vi "XY stage App.vi"() -> ()   [LabVIEW 2017]
uses:
  Newport.XPS.CommandInterface
panel:
  in  "Stop Program":bool
  in  "Start Program":bool
  in  "Move Inverse":bool
  in  "Move Normal":bool
  out "Expected Output":cluster{"X":dbl, "Y":dbl}[](graph)
  out "Total Time Horizontal":dbl
  out "Total Time Vertical":dbl
  in  "Velocity and Acceleration Input":cluster{"Velocity":dbl, "Acceleration":dbl}={"Velocity"=150.0, "Acceleration"=2000.0} {"Acceleration" min=0.0; "Velocity" min=0.0}
  in  "Abort Motion":bool
  out "Total Y Path":dbl
  in  "Absolute Target 2":cluster{"X Position":dbl, "Y Position":dbl}[](array[cluster]) {"Y Position" min=-100.0 max=100.0; "X Position" min=-100.0 max=100.0}
  in  "Start Absolute 2":bool
  out "Current Y Position":dbl[](array[numeric])
  out "Current X Position":dbl[](array[numeric])
  out "Total X Path":dbl
  in  "Number of Horizontal Sections":u32
  in  "Number of Vertical Sections":u32
  in  "Horizontal Segments Parameters":T1(array[cluster]) {"velocity" min=0.0; "Y rel dist" min=-100.0 max=100.0; "X rel dist" min=-100.0 max=100.0}
  in  "Vertical Segments Parameters":T1(array[cluster]) {"velocity" min=0.0; "Y rel dist" min=-100.0 max=100.0; "X rel dist" min=-100.0 max=100.0}
  in  "Absolute Target 1":cluster{"X Position":dbl, "Y Position":dbl}[](array[cluster]) {"Y Position" min=-100.0 max=100.0; "X Position" min=-100.0 max=100.0}
  in  "Start Absolute 1":bool
  in  "Go Home":bool
  in  "Kill All":bool
  # "Absolute Movement"
  # "Relative Movement"
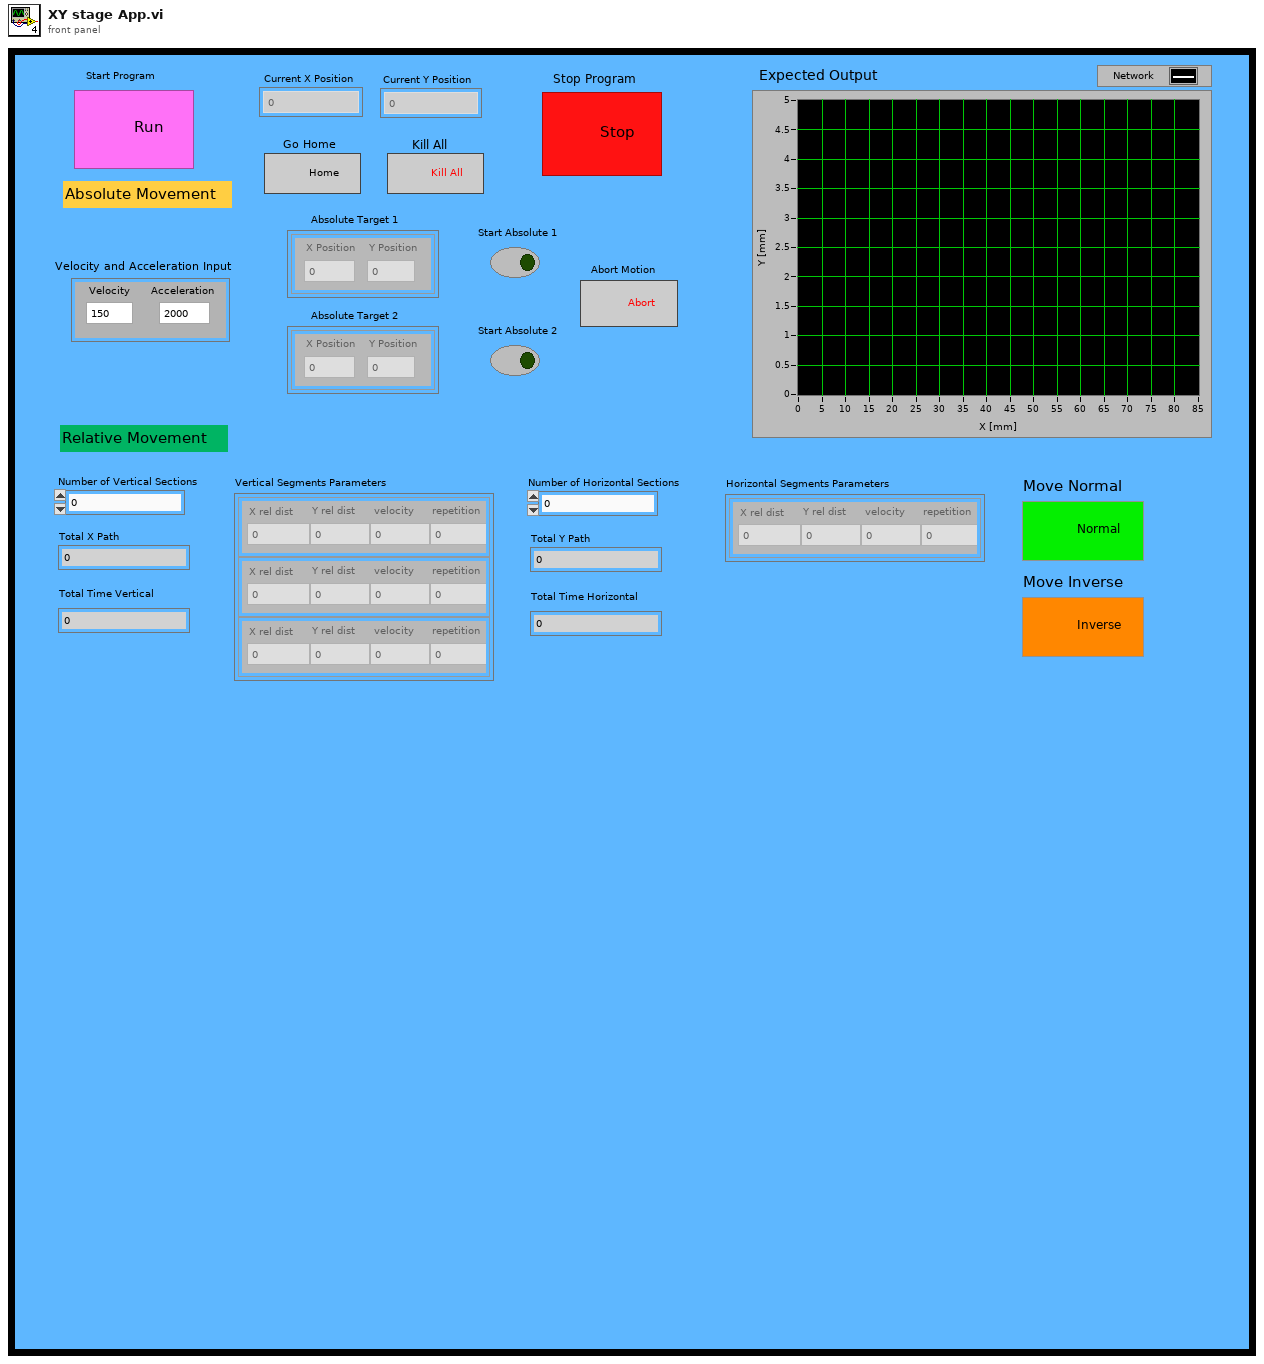
[diagram p1: front panel]
types:
  T1 = cluster{"X rel dist":dbl, "Y rel dist":dbl, "velocity":dbl, "repetition":u32}[]
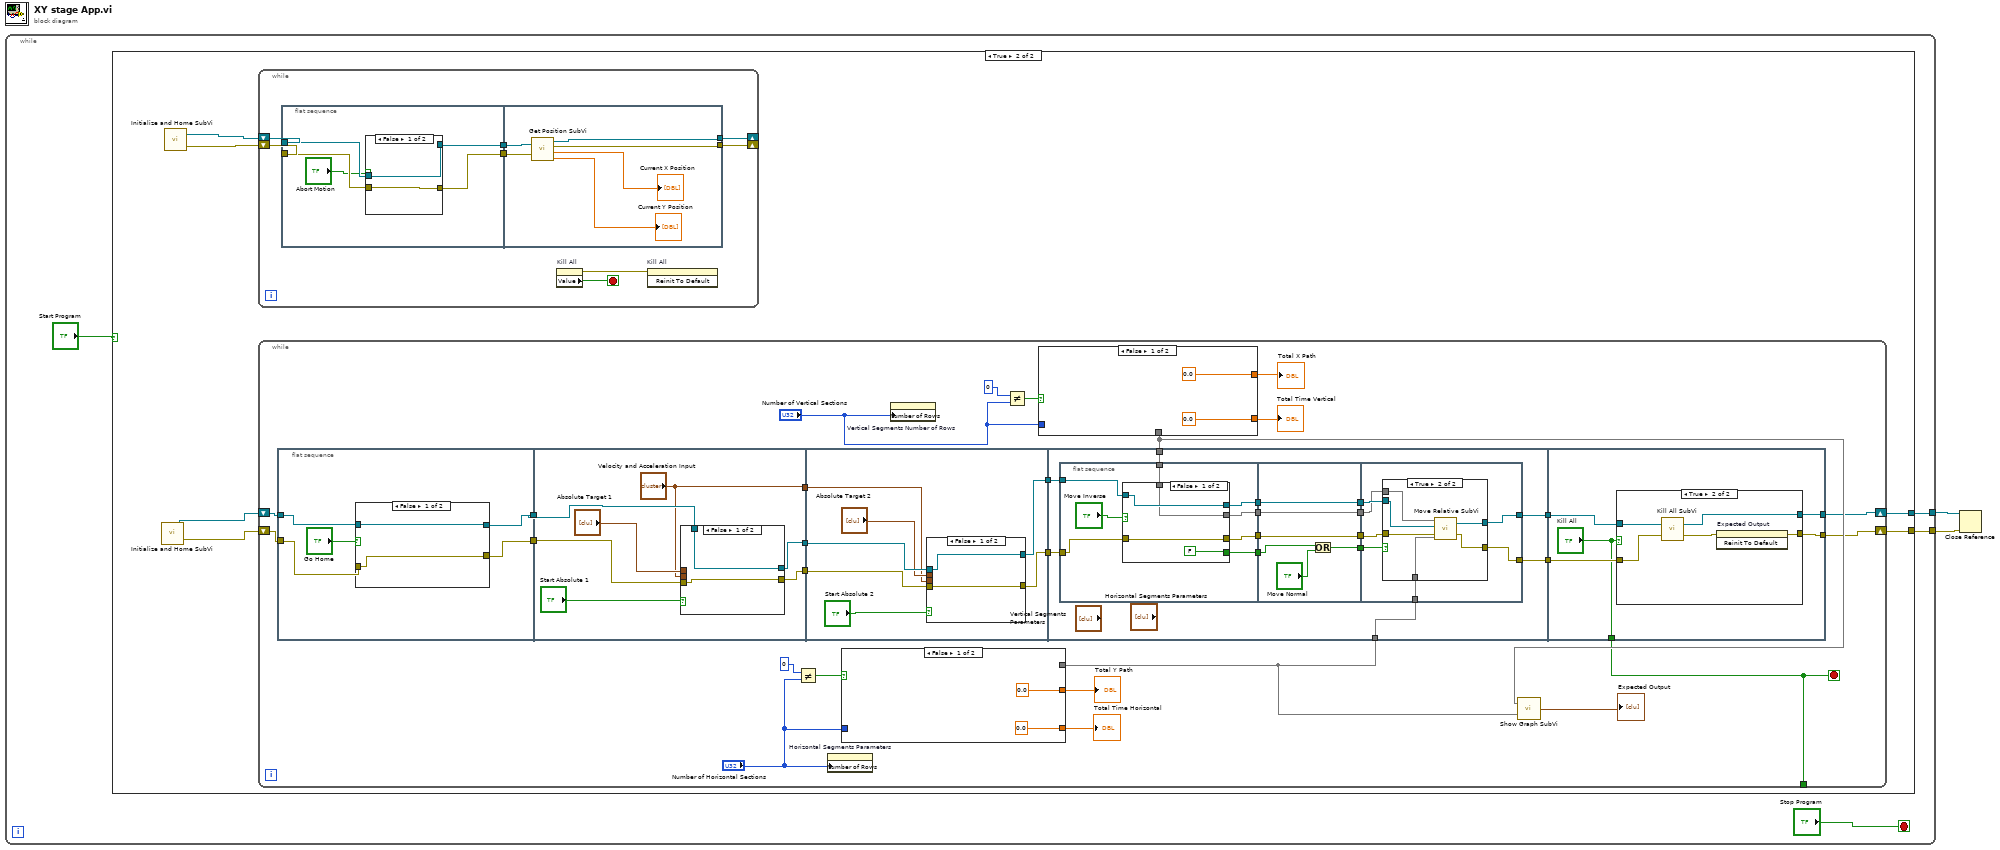
[diagram p0: block diagram]
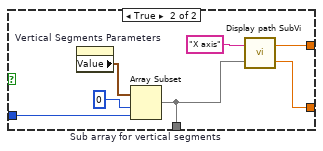
[diagram p3: hidden frame]
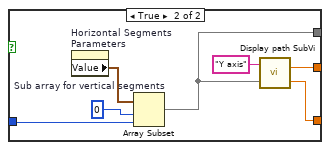
[diagram p4: hidden frame]
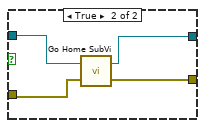
[diagram p5: hidden frame]
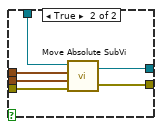
[diagram p6: hidden frame]
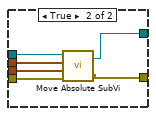
[diagram p7: hidden frame]
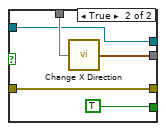
[diagram p8: hidden frame]
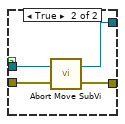
[diagram p11: hidden frame]
diagram:
  n1 = while {
    tunnel: [w6] -> w1
    tunnel: [w5] -> w2
    stop <- "Stop Program" stop-if-true
    n2 = case shown="True" "Start Program" {
      tunnel: [_ w8] -> w6
      tunnel: [_ w7] -> w5
      frame False {
      }
      frame True {
        n3 = call "Initialize and Home SubVi.vi"() -> ("error out"=w11:errorcluster, "reference out"=w12:refnum<k24>)  [unwired: 2 in]
        n4 = call "Initialize and Home SubVi.vi"() -> ("error out"=w9:errorcluster, "reference out"=w10:refnum<k24>)  [unwired: 2 in]
        n5 = while {
          shift-right: [w170] -> _
          shift-left: w10 -> [w168]
          shift-right: [w169] -> _
          shift-left: w9 -> [w167]
          stop <- w164 stop-if-true
          n6 = flat-sequence {
            tunnel: w167 -> [w173]
            tunnel: w168 -> [w174]
            tunnel: [w175] -> w166
            tunnel: [w172] -> w165
            tunnel: [w187] -> w170
            tunnel: [w186] -> w169
            tunnel: w166 -> [w183]
            tunnel: w165 -> [w182]
            frame #0 {
              n7 = case shown="False" "Abort Motion" {
                tunnel: [w177 w180] -> w175
                tunnel: w174 -> [w177 w181]
                tunnel: w173 -> [w176 w179]
                tunnel: [w176 w178] -> w172
                frame False {
                }
                frame True {
                  n8 = call "Abort Move SubVi.vi"("error in"=w179, "reference in"=w181) -> ("error out"=w178:errorcluster, "reference out"=w180:refnum<k24>)
                }
              }
            }
            frame #1 {
              n9 = call "Get Position SubVi.vi"("reference in"=w183, "error in"=w182) -> ("reference out"=w187:refnum<k24>, "error out"=w186:errorcluster, "Current X Position"=→"Current X Position":dbl[], "Current Y Position"=→"Current Y Position":dbl[])
            }
          }
          n10 = property on="Kill All" class="Bool (strict)"() -> (error out=w163:errorcluster, "Value"=w164:bool)  [unwired: 2 in, 1 out]
          n11 = invoke on="Kill All" class="Bool (strict)" method="Reinit To Default"(error in=w163) -> ()  [unwired: 2 in, 3 out]
        }
        n12 = while {
          shift-right: [w15] -> w8
          shift-left: w12 -> [w39]
          shift-right: [w14] -> w7
          shift-left: w11 -> [w38]
          tunnel: [w13] -> _
          stop <- w13 stop-if-true
          n13 = flat-sequence {
            tunnel: w39 -> [w58]
            tunnel: [w59] -> w37
            tunnel: w38 -> [w61]
            tunnel: [w62] -> w36
            tunnel: w37 -> [w75]
            tunnel: w36 -> [w73]
            tunnel: [w71] -> w35
            tunnel: [w70] -> w33
            tunnel: ["Velocity and Acceleration Input"] -> w29
            tunnel: w35 -> [w87]
            tunnel: [w88] -> w34
            tunnel: w33 -> [w90]
            tunnel: [w89] -> w32
            tunnel: w29 -> [w85]
            tunnel: [w101] -> w31
            tunnel: w34 -> [w111]
            tunnel: [w102] -> w30
            tunnel: w32 -> [w110]
            tunnel: w27 -> [w112]
            tunnel: w16 -> [w103]
            tunnel: ["Kill All"] -> w13
            tunnel: w30 -> [w154]
            tunnel: w31 -> [w155]
            tunnel: [w153] -> w15
            tunnel: [w152] -> w14
            frame #0 {
              n14 = case shown="False" "Go Home" {
                tunnel: [w63 w68] -> w62
                tunnel: w61 -> [w63 w67]
                tunnel: [w64 w66] -> w59
                tunnel: w58 -> [w64 w65]
                frame False {
                }
                frame True {
                  n15 = call "Go Home SubVi.vi"("error in"=w67, "reference in"=w65) -> ("error out"=w68:errorcluster, "reference out"=w66:refnum<k24>)
                }
              }
            }
            frame #1 {
              n16 = case shown="False" "Start Absolute 1" {
                tunnel: w75 -> [w76 w83]
                tunnel: "Absolute Target 1" -> [_ w82]
                tunnel: w73 -> [w77 w81]
                tunnel: "Velocity and Acceleration Input" -> [_ w80]
                tunnel: [w76 w79] -> w71
                tunnel: [w77 w78] -> w70
                frame False {
                }
                frame True {
                  n17 = call "Move Absolute SubVi.vi"("error in"=w81, "Vel and Acc"=w80, "Absolute Movement"=w82, "reference in"=w83) -> ("error out"=w78:errorcluster, "reference out"=w79:refnum<k24>)
                }
              }
            }
            frame #2 {
              n18 = case shown="False" "Start Absolute 2" {
                tunnel: w90 -> [w91 w98]
                tunnel: [w91 w97] -> w89
                tunnel: [w92 w96] -> w88
                tunnel: w87 -> [w92 w95]
                tunnel: "Absolute Target 2" -> [_ w94]
                tunnel: w85 -> [_ w93]
                frame False {
                }
                frame True {
                  n19 = call "Move Absolute SubVi.vi"("error in"=w98, "Vel and Acc"=w93, "Absolute Movement"=w94, "reference in"=w95) -> ("error out"=w97:errorcluster, "reference out"=w96:refnum<k24>)
                }
              }
            }
            frame #3 {
              n20 = flat-sequence {
                tunnel: w112 -> [w114]
                tunnel: w111 -> [w118]
                tunnel: w110 -> [w116]
                tunnel: [w120] -> w109
                tunnel: [w117] -> w108
                tunnel: [w115] -> w107
                tunnel: [w113] -> w100
                tunnel: w109 -> [w135]
                tunnel: w108 -> [w134]
                tunnel: w107 -> [w133]
                tunnel: [w135] -> w106
                tunnel: [w134] -> w105
                tunnel: [w133] -> w104
                tunnel: w100 -> [w132]
                tunnel: [w130] -> w99
                tunnel: w106 -> [w140]
                tunnel: w105 -> [w142]
                tunnel: w104 -> [w141]
                tunnel: w103 -> [w139]
                tunnel: [w138] -> w102
                tunnel: [w137] -> w101
                tunnel: w99 -> [w136]
                frame #0 {
                  n21 = case shown="False" "Move Inverse" {
                    tunnel: [w121 w129] -> w120
                    tunnel: [FALSE TRUE] -> w113
                    tunnel: w114 -> [w121 w127]
                    tunnel: w118 -> [w124 w126]
                    tunnel: [w124 w126] -> w117
                    tunnel: w116 -> [w123 w125]
                    tunnel: [w123 w125] -> w115
                    frame False {
                    }
                    frame True {
                      n22 = call "Change X Direction.vi"("Vertical Segments Parameters in"=w127) -> ("Vertical Segments Parameters out"=w129:T1)
                    }
                  }
                }
                frame #1 {
                  n23 = Or(x=w132, y="Move Normal") -> (x .or. y?=w130:bool)
                }
                frame #2 {
                  n24 = case shown="True" w136 {
                    tunnel: w142 -> [w144 w150]
                    tunnel: w141 -> [w143 w146]
                    tunnel: [w143 w145] -> w138
                    tunnel: [w144 w147] -> w137
                    tunnel: w140 -> [_ w148]
                    tunnel: w139 -> [_ w149]
                    frame False {
                    }
                    frame True {
                      n25 = call "Move Relative SubVi.vi"("Horizontal Segments Parameters"=w149, "error in"=w146, "reference in"=w150, "Vertical Segments Parameters"=w148) -> ("error in 2"=w145:errorcluster, "reference out"=w147:refnum<k24>)
                    }
                  }
                }
              }
            }
            frame #4 {
              n26 = case shown="True" "Kill All" {
                tunnel: w155 -> [w157 w159]
                tunnel: w154 -> [w156 w158]
                tunnel: [w157 w162] -> w153
                tunnel: [w156 w160] -> w152
                frame False {
                }
                frame True {
                  n27 = call "Kill All SubVi.vi"("error in"=w158, "reference in"=w159) -> ("error out"=w161:errorcluster, "reference out"=w162:refnum<k24>)
                  n28 = invoke on="Expected Output" class="XYGraph (strict)" method="Reinit To Default"(error in=w161) -> (error out=w160:errorcluster)  [unwired: 2 in, 2 out]
                }
              }
            }
          }
          n29 = Not Equal?(x=0, y="Number of Horizontal Sections") -> (x != y?=w22:bool)
          n30 = property on="Horizontal Segments Parameters" class="Arr (strict)"("Number of Rows"="Number of Horizontal Sections") -> ()  [unwired: 2 in, 2 out]
          n31 = case shown="False" w22 {
            tunnel: [_ w55] -> w16
            tunnel: "Number of Horizontal Sections" -> [_ w54]
            tunnel: [0.0 ("Total Time") w51] -> w20
            tunnel: [0.0 ("Total Path") w52] -> w19
            frame False {
            }
            frame True {
              n32 = property on="Horizontal Segments Parameters" class="Arr (strict)"() -> ("Value"=w56:T1)  [unwired: 2 in, 2 out]
              n33 = Array Subset "Sub array for vertical segments"(array=w56, index=0, length=w54) -> (w55:T1)
              n34 = call "Display path SubVi.vi"("Array"=w55, "Combo Box"="Y axis") -> ("Total Time"=w51:dbl, "Total Path"=w52:dbl)
            }
          }
          "Total Y Path" <- w19
          "Total Time Horizontal" <- w20
          n35 = property on="Vertical Segments Number of Rows" class="Arr (strict)"("Number of Rows"="Number of Vertical Sections") -> ()  [unwired: 2 in, 2 out]
          n36 = Not Equal?(x=u32 0, y="Number of Vertical Sections") -> (x != y?=w21:bool)
          n37 = case shown="False" w21 {
            tunnel: [_ w46] -> w27
            tunnel: "Number of Vertical Sections" -> [_ w45]
            tunnel: [0.0 ("Total Path") w43] -> w18
            tunnel: [0.0 ("Total Time") w42] -> w17
            frame False {
            }
            frame True {
              n38 = property on="Vertical Segments Parameters" class="Arr (strict)"() -> ("Value"=w47:T1)  [unwired: 2 in, 2 out]
              n39 = Array Subset "Sub array for vertical segments"(array=w47, index=0, length=w45) -> (w46:T1)
              n40 = call "Display path SubVi.vi"("Array"=w46, "Combo Box"="X axis") -> ("Total Time"=w42:dbl, "Total Path"=w43:dbl)
            }
          }
          "Total X Path" <- w18
          "Total Time Vertical" <- w17
          n41 = call "Show Graph SubVi.vi"("Horizontal Segments Parameters"=w16, "Vertical Segments Parameters"=w27) -> ("Output Array"=→"Expected Output":cluster{"X":dbl, "Y":dbl}[])
        }
      }
    }
  }
  n42 = Close Reference(reference=w1, error in (no error)=w2) -> ()  [unwired: 1 out]
